vi "Process Mouse Down.vi"(0 "FSM.Graph in":T1, 5 "Display State In":T2, 7 "Coords":T3, 9 "PlatMods":T6, 11 "Editor Ref":refnum<vi>) -> (4 "FSM.Graph out":T1, 6 "Display State Out":T2)   [LabVIEW 2015, in "FSM Editor.xctl"]
uses:
  FSM Editor.xctl
  <vilib>/Utility/miscctls.llb/LVPoint32TypeDef.ctl
  State.vi
  Classes/FSM.Port/FSM.Port.lvclass
  Drag Mode.ctl
  Events.ctl
  NodeAdded.ctl
  NodeSelected.ctl
  EdgeEventData.ctl
  Data.vi
  Classes/FSM.Graph/FSM.Graph.lvclass
  <vilib>/Utility/cursorutil.llb/Set Cursor (Icon Pict).vi
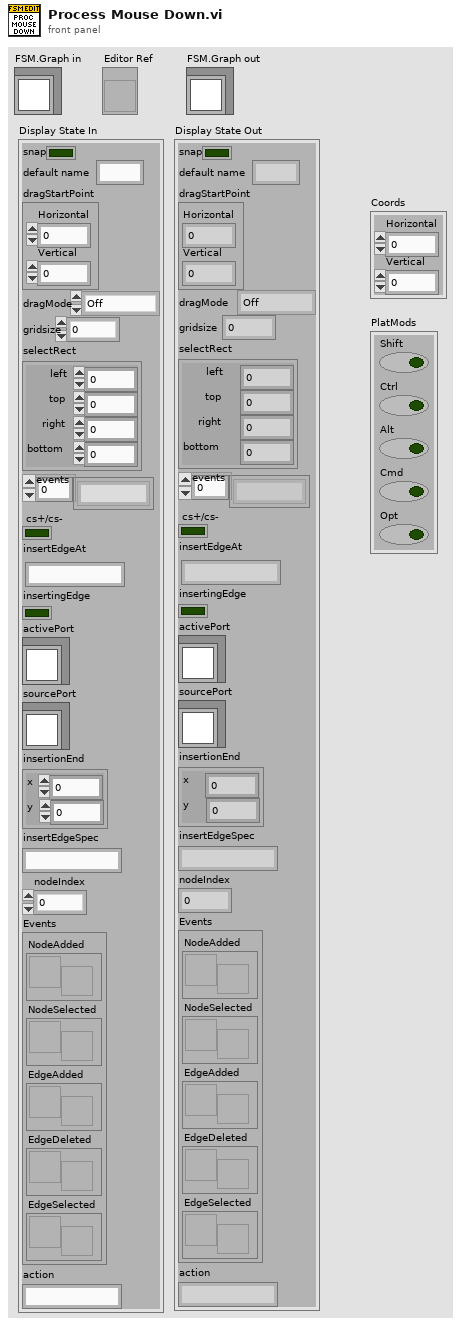
[diagram p1: front panel]
types:
  T1 = typedef "FSM Editor.xctl/Data.vi" = refnum<class "FSM.Graph.lvclass">
  T2 = typedef "FSM Editor.xctl/State.vi" = cluster{"snap":bool, "default name":string, "dragStartPoint":T3, "dragMode":T4, "gridsize":dbl, "selectRect":cluster{"left":i16, "top":i16, "right":i16, "bottom":i16}, "events":string[], "cs+/cs-":bool, "insertEdgeAt":string, "insertingEdge":bool, "activePort":refnum<class "FSM.Port.lvclass">, "sourcePort":refnum<class "FSM.Port.lvclass">, "insertionEnd":cluster{"x":i16, "y":i16}, "insertEdgeSpec":string, "nodeIndex":i32, "Events":T5, "action":string}
  T3 = typedef "LVPoint32TypeDef.ctl" = cluster{"Horizontal":i32, "Vertical":i32}
  T4 = typedef "Drag Mode.ctl" = enum16{"Off", "NodePending", "Nodes", "Pan", "Select", "EdgeInsertion", "EdgePoint", "EdgeLabel"}
  T5 = typedef "FSM Editor.xctl/Events.ctl" = cluster{"NodeAdded":refnum<user-event>, "NodeSelected":refnum<user-event>, "EdgeAdded":refnum<user-event>, "EdgeDeleted":refnum<user-event>, "EdgeSelected":refnum<user-event>}
  T6 = cluster{"Shift":bool, "Ctrl":bool, "Alt":bool, "Cmd":bool, "Opt":bool}
  T7 = enum16{"Off", "NodePending", "Nodes", "Pan", "Select", "EdgeInsertion", "EdgePoint", "EdgeLabel"}
  T8 = cluster{"left":i16, "top":i16, "right":i16, "bottom":i16}
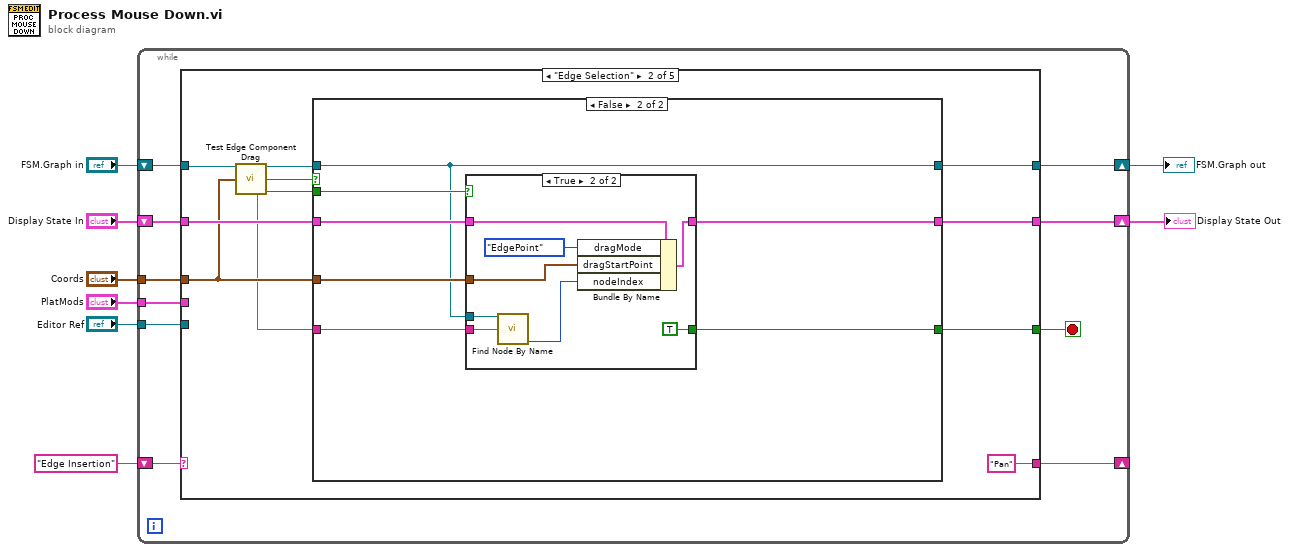
[diagram p0: block diagram]
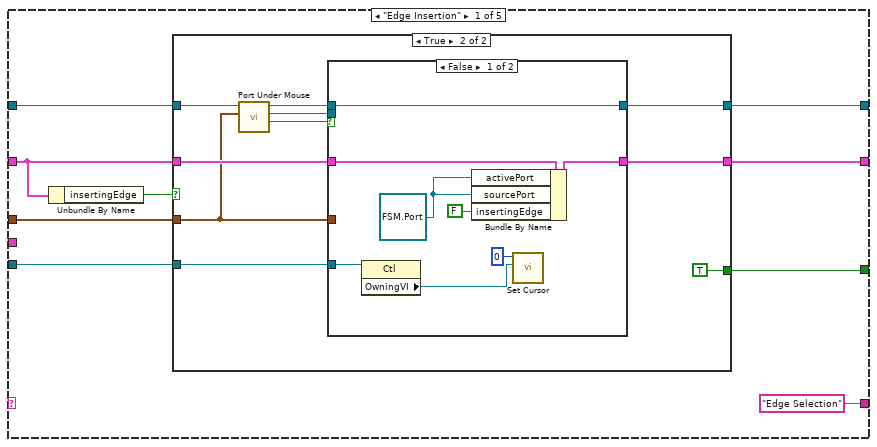
[diagram p2: hidden frame]
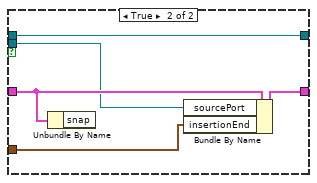
[diagram p4: hidden frame]
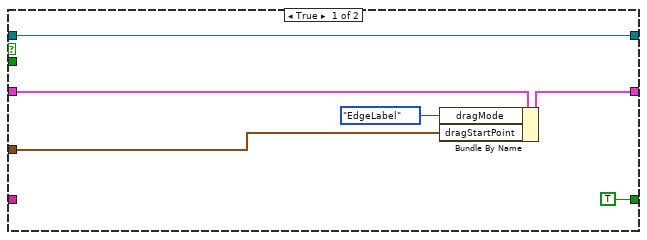
[diagram p5: hidden frame]
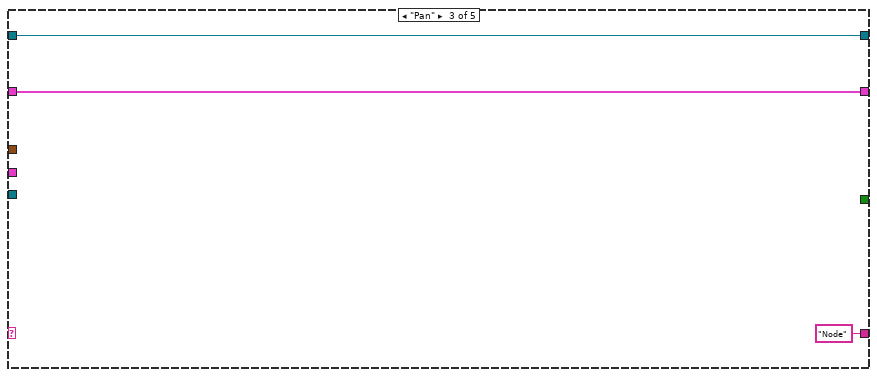
[diagram p7: hidden frame]
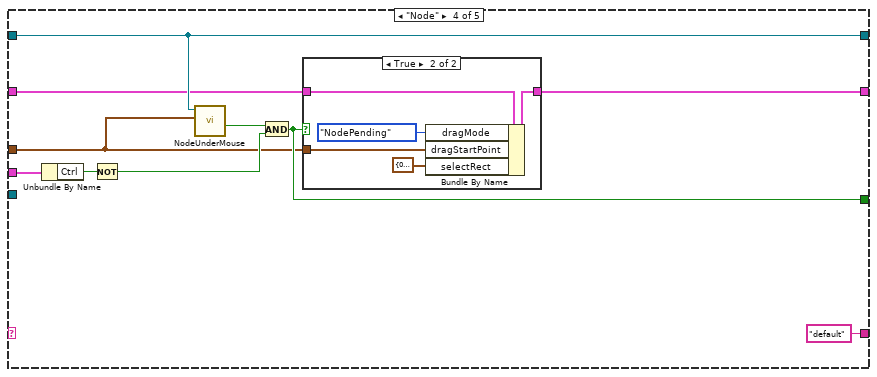
[diagram p8: hidden frame]
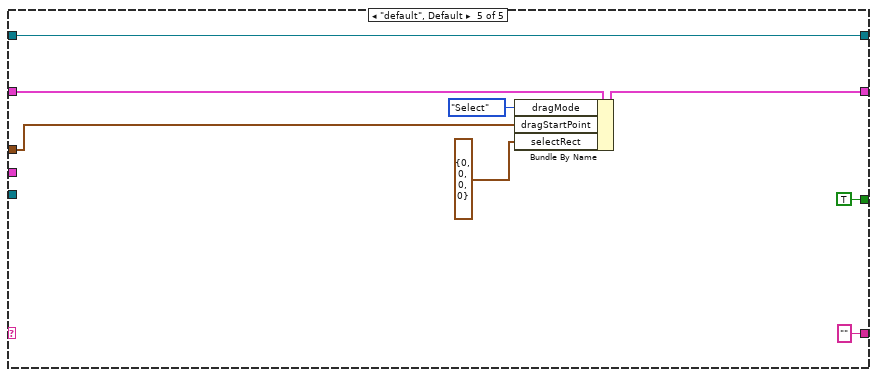
[diagram p10: hidden frame]
diagram:
  n1 = while {
    shift-right: [w16] -> w7
    shift-left: "FSM.Graph in" -> [w15]
    shift-right: [w17] -> _
    shift-left: "Edge Insertion" -> [w18]
    tunnel: "Coords" -> [w13]
    tunnel: "PlatMods" -> [w12]
    shift-right: [w11] -> w2
    shift-left: "Display State In" -> [w14]
    tunnel: "Editor Ref" -> [w9]
    stop <- w10 stop-if-true
    n2 = case shown="\"Edge Selection\"" w18 {
      tunnel: ["Edge Selection" "Pan" "Node" "default" ""] -> w17
      tunnel: [w23 w61 w87 w98 w112] -> w16
      tunnel: w15 -> [w24 w59 w87 w98 w112]
      tunnel: w14 -> [w26 w62 w86 w92 w111]
      tunnel: w13 -> [w21 w55 _ w89 w109]
      tunnel: w12 -> [_ _ _ w96 _]
      tunnel: [w22 w60 w86 w91 w110] -> w11
      tunnel: [w20 w56 _ w90 TRUE] -> w10
      tunnel: w9 -> [w19 _ _ _ _]
      frame "Edge Insertion" {
        n3 = Unbundle By Name(w26) -> ("insertingEdge"=w25:bool)
        n4 = case shown="True" w25 {
          tunnel: w26 -> [w28 w35]
          tunnel: w24 -> [w29 w39]
          tunnel: [w29 w34] -> w23
          tunnel: [w28 w33] -> w22
          tunnel: w21 -> [_ w30]
          tunnel: [_ TRUE] -> w20
          tunnel: w19 -> [_ w31]
          frame False {
          }
          frame True {
            n5 = call "Port Under Mouse.vi"("point"=w30, "FSM in"=w39) -> ("found?"=w37:bool, "Port"=w36:refnum<class "FSM.Port.lvclass">, "FSM out"=w38:T1)  [unwired: 6 in, 1 out]
            n6 = case shown="False" w37 {
              tunnel: w38 -> [w47 w52]
              tunnel: w36 -> [_ w49]
              tunnel: w35 -> [w46 w51]
              tunnel: [w47 w52] -> w34
              tunnel: [w45 w50] -> w33
              tunnel: w31 -> [w41 _]
              tunnel: w30 -> [_ w48]
              frame False {
                w44 = refnum<class "FSM.Port.lvclass"> refnum ("FSM.Port")
                n7 = property class="Ctl"(reference=w41) -> ("OwningVI"=w40:refnum<vi>)  [unwired: 1 in, 2 out]
                n8 = Bundle By Name(cluster=w46, "activePort"=w44, "sourcePort"=w44, "insertingEdge"=FALSE) -> (w45:T2)
                n9 = call-poly <vilib>:"Set Cursor.vi"("VI reference (current VI)"=w40, "icon"=u16 0) -> ()  [unwired: 8 in, 2 out]
              }
              frame True {
                n10 = Unbundle By Name(w51) -> ()  [unwired: 1 out]
                n11 = Bundle By Name(cluster=w51, "sourcePort"=w49, "insertionEnd"=w48) -> (w50:T2)
              }
            }
          }
        }
      }
      frame "Edge Selection" {
        n12 = call "Test Edge Component Drag.vi"("FSM.Graph In"=w59, "Coords"=w55) -> ("FSM.Graph Out"=w58:T1, "label drag?"=w57:bool, "attached node"=w53:string, "drag control?"=w54:bool)  [unwired: 10 in]
        n13 = case shown="False" w57 {
          tunnel: w58 -> [w69 w71]
          tunnel: w62 -> [w68 w75]
          tunnel: [w69 w71] -> w61
          tunnel: [w67 w73] -> w60
          tunnel: [TRUE w70] -> w56
          tunnel: w55 -> [w64 w74]
          tunnel: w54 -> [_ w76]
          tunnel: w53 -> [_ w72]
          frame True {
            n14 = Bundle By Name(cluster=w68, "dragMode"=T7."EdgeLabel", "dragStartPoint"=w64) -> (w67:T2)
          }
          frame False {
            n15 = case shown="True" w76 {
              tunnel: w75 -> [w77 w85]
              tunnel: w74 -> [_ w83]
              tunnel: [w77 w82] -> w73
              tunnel: w72 -> [_ w81]
              tunnel: w71 -> [_ w80]
              tunnel: [_ TRUE] -> w70
              frame False {
              }
              frame True {
                n16 = call "Find Node By Name.vi"("FSM.Graph"=w80, "Name"=w81) -> ("index"=w79:i32)  [unwired: 12 in, 1 out]
                n17 = Bundle By Name(cluster=w85, "dragMode"=Drag_Mode."EdgePoint", "dragStartPoint"=w83, "nodeIndex"=w79) -> (w82:T2)
              }
            }
          }
        }
      }
      frame "Pan" {
      }
      frame "Node" {
        n18 = Unbundle By Name(w96) -> ("Ctrl"=w95:bool)
        n19 = Not(x=w95) -> (.not. x?=w94:bool)
        n20 = call "NodeUnderMouse.vi"("Coords"=w89, "FSM in"=w98) -> ("contains mouse"=w97:bool)  [unwired: 6 in, 3 out]
        n21 = And(x=w97, y=w94) -> (x .and. y?=w90:bool)
        n22 = case shown="True" w90 {
          tunnel: w92 -> [w99 w104]
          tunnel: [w99 w103] -> w91
          tunnel: w89 -> [_ w102]
          frame False {
          }
          frame True {
            n23 = Bundle By Name(cluster=w104, "dragMode"=Drag_Mode."NodePending", "dragStartPoint"=w102, "selectRect"=T8 {"left"=0, "top"=0, "right"=0, "bottom"=0}) -> (w103:T2)
          }
        }
      }
      frame "default", Default {
        n24 = Bundle By Name(cluster=w111, "dragMode"=T7."Select", "dragStartPoint"=w109, "selectRect"=T8 {"left"=0, "top"=0, "right"=0, "bottom"=0}) -> (w110:T2)
      }
    }
  }
  "Display State Out" <- w2
  "FSM.Graph out" <- w7
